vi "Example with Results.vi"(3 "Table Content":T1={"TableHeader"=["Soll\nppm/%", "Ist\nppm/%", "Fehler\n%", "Toleranz\n%", "Ergebnis"], "Table"=[["aaa", "bbb", "ccc", "ddd"], ["111", "222", "333", "444"], ["sss", "fff", "kkk", "xxx"], ["6.5", "11.13", "19.2", "4"], ["1111", "1212", "777", "888"]], "Relative Column Widths (%)"=[22.5, 22.5, 22.5, 22.5, 10.0], "Results"=[{"Result Text"="ok", "Result"=TRUE}, {"Result Text"="ko", "Result"=FALSE}, {"Result Text"="ko", "Result"=FALSE}, {"Result Text"="ok", "Result"=TRUE}, {"Result Text"="ok", "Result"=TRUE}], "PositionBemerkung"=enum."before", "PageBreak"=enum."before"}) -> (11 "XY-Graph":cluster{"X":dbl, "Y":dbl}[](graph))   [LabVIEW 2020, in "PDF Interface.lvlib"]
uses:
  PDF Interface.lvlib
  <vilib>/Simplicity AI/SAI_PDF_API/Classes/Context/Controls/SAI_PDF_Text Align.ctl
  <vilib>/Simplicity AI/SAI_PDF_API/Classes/Context/Context.lvclass
  <vilib>/Simplicity AI/SAI_PDF_API/Classes/Context/Controls/SAI_PDF_PDF Details.ctl
  PDF Interface Helper/PDFTableContentType.ctl
  PDF Interface Helper/PDF Interface Helper.lvlib
  PDF Interface Helper/PDFContentType.ctl
  PDF Interface Helper/PDFPageBreak.ctl
  PDF Interface Helper/PDFCommentPosition.ctl
  PDF Interface Helper/PDFTablePictures.ctl
  PDF Interface Helper/PDFResultPictures.ctl
  PDF Interface Helper/PDFResults.ctl
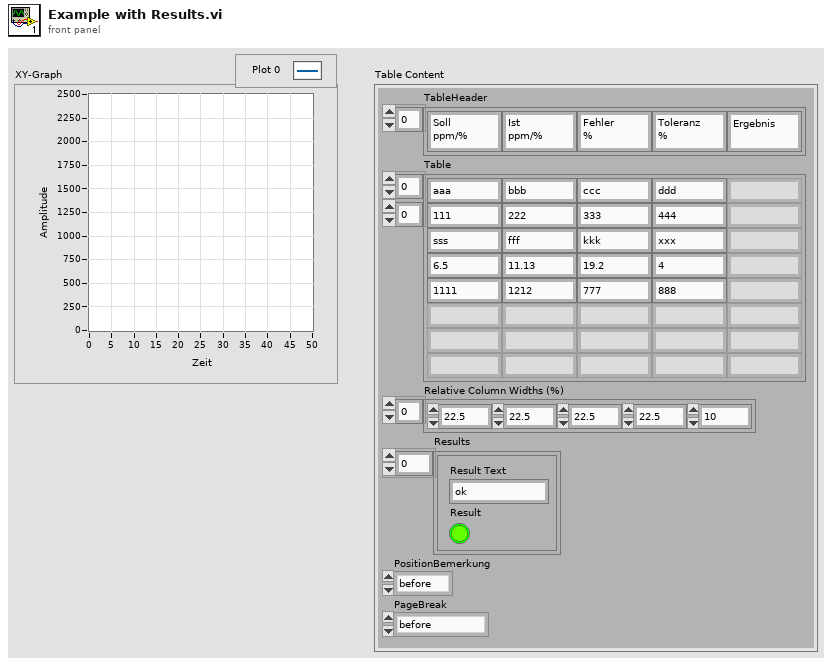
[diagram p1: front panel]
types:
  T1 = typedef "PDF Interface.lvlib/PDF Interface Helper.lvlib/PDFTableContentType.ctl" = cluster{"TableHeader":string[], "Table":string[][], "Relative Column Widths (%)":sgl[], "Results":cluster{"Result Text":string, "Result":bool}[], "PositionBemerkung":T2, "PageBreak":T3}
  T2 = typedef "PDF Interface.lvlib/PDF Interface Helper.lvlib/PDFCommentPosition.ctl" = enum16{"before", "after"}
  T3 = typedef "PDF Interface.lvlib/PDF Interface Helper.lvlib/PDFPageBreak.ctl" = enum16{"none", "before", "after", "after comment"}
  T4 = typedef "PDF Interface.lvlib/PDF Interface Helper.lvlib/PDFContentType.ctl" = cluster{"Titel":string, "Header Table":string[][], "Table Array":T5[], "Bemerkungen":cluster{"Bemerkung Text":string, "Align (Left)":T9, "Add Line Feeds (F:No)":bool}[]}
  T5 = typedef "PDF Interface.lvlib/PDF Interface Helper.lvlib/PDFTableContentType.ctl" = cluster{"TableHeader":string[], "Table":string[][], "Relative Column Widths (%)":sgl[], "Results":T6, "PositionBemerkung":T2, "PageBreak":T3, "TablePictures":T8, "Horizontal Align":i32}
  T6 = typedef "PDF Interface.lvlib/PDF Interface Helper.lvlib/PDFResults.ctl" = cluster{"Results":cluster{"Result Text":string, "Result":bool}[], "ResultPictures":T7, "use Pictures":bool}
  T7 = typedef "PDF Interface.lvlib/PDF Interface Helper.lvlib/PDFResultPictures.ctl" = cluster{"Yes Ctl Refnum":refnum<vi>, "No Ctl Refnum":refnum<vi>}
  T8 = typedef "PDF Interface.lvlib/PDF Interface Helper.lvlib/PDFTablePictures.ctl" = cluster{"Ctl Refnum In":refnum<vi>[], "RowOrColumn":enum16{"Row", "Column"}, "IndexToInsert":u16, "Image Scale (%)":sgl[], "Autoscale? (T)":bool[], "Horizontal Align":i32}
  T9 = typedef "SAI_PDF_Toolkit.lvlib/Context.lvclass/SAI_PDF_Text Align.ctl" = i32
  T10 = cluster{"Bemerkung Text":string, "Align (Left)":T9, "Add Line Feeds (F:No)":bool}[]
  T11 = cluster{"GraphCtl Refnum":refnum<vi>, "Wrap Text (F:No)":bool, "Hide Grid (F:No)":bool, "Scale (100%)":sgl, "Align (Left)":T9}
  T12 = typedef "SAI_PDF_Toolkit.lvlib/Context.lvclass/SAI_PDF_PDF Details.ctl" = cluster{"Title":string, "Subject":string, "Keywords":string, "Author":string, "Creator":string}
  T13 = cluster{"Header Footer Text Cluster":cluster{"Header Text":string, "Footer Text":string, "Time":string, "Page Number":string}, "PDF Details":T12}
  T14 = cluster{"GraphCtl Refnum":refnum<vi>, "Wrap Text (F:No)":bool, "Hide Grid (F:No)":bool, "Scale (100%)":sgl, "Align (Left)":T9}[]
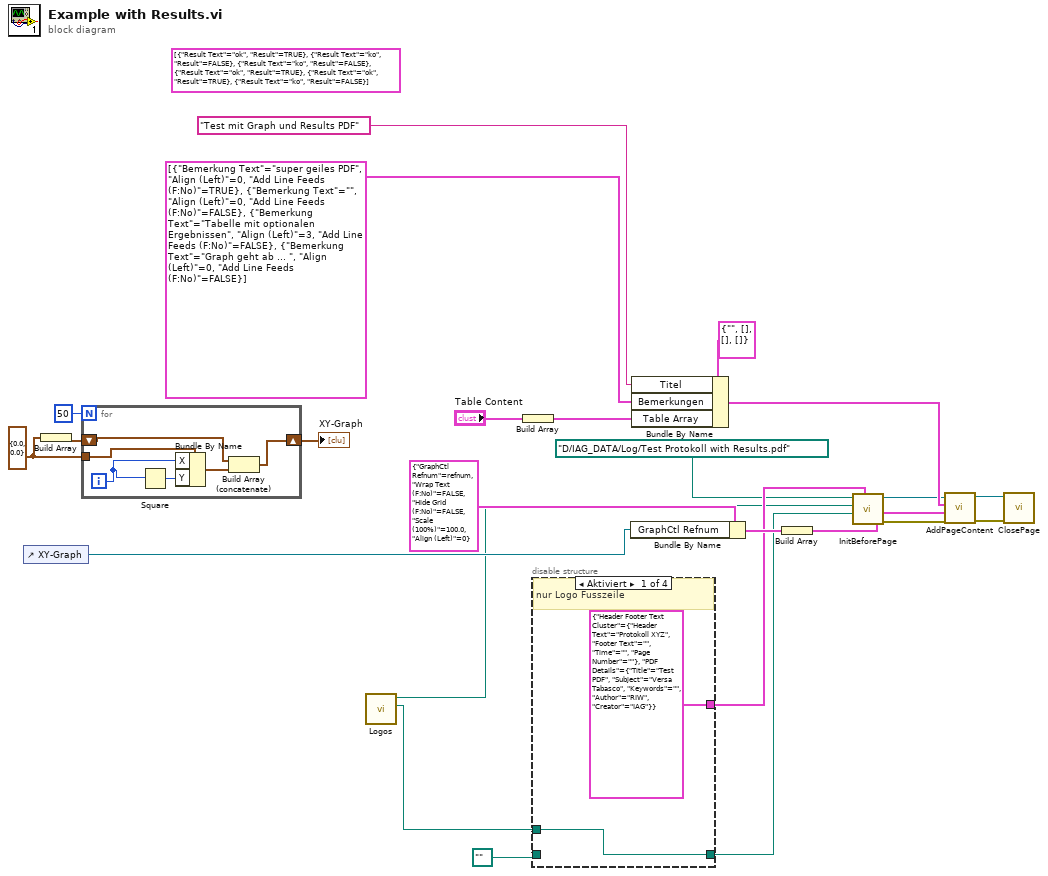
[diagram p0: block diagram]
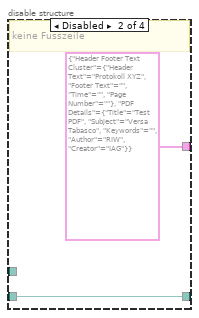
[diagram p2: hidden frame]
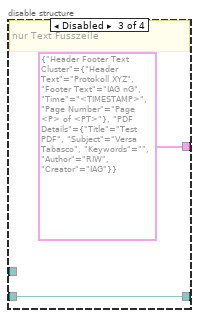
[diagram p3: hidden frame]
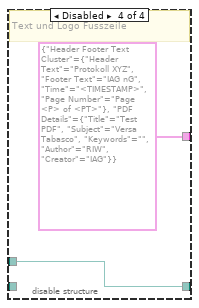
[diagram p4: hidden frame]
diagram:
  (unwired) cluster{"Result Text":string, "Result":bool}[] [{"Result Text"="ok", "Result"=TRUE}, {"Result Text"="ko", "Result"=FALSE}, {"Result Text"="ko", "Result"=FALSE}, {"Result Text"="ok", "Result"=TRUE}, {"Result Text"="ok", "Result"=TRUE}, {"Result Text"="ko", "Result"=FALSE}] ("Results")
  w21 = cluster{"X":dbl, "Y":dbl} {"X"=0.0, "Y"=0.0} ("XY-Graph")
  n1 = control-ref of="XY-Graph"() -> (w18:refnum<vi>)
  n2 = Build Array(w21) -> (w22:cluster{"X":dbl, "Y":dbl}[])
  n3 = for {
    N: 50 -> [_]
    shift-right: [w25] -> w23
    shift-left: w22 -> [w27]
    tunnel: w21 -> [w26]
    i -> [w29]
    n4 = Square(x=w29) -> (x^2=w30:i32)
    n5 = Bundle By Name(cluster=w26, "X"=w29, "Y"=w30) -> (w28:cluster{"X":dbl, "Y":dbl})
    n6 = Build Array (concatenate)(w27, w28) -> (w25:cluster{"X":dbl, "Y":dbl}[])
  }
  "XY-Graph" <- w23
  n7 = call "Logos.vi"() -> ("Footer Image File Path"=w13:path, "Header Image File Path"=w10:path)  [unwired: 9 in, 1 out]
  n8 = Build Array("Table Content") -> (w1:T1[])
  n9 = disable-structure shown="Aktiviert" {
    disable-tunnel: [T13 {"Header Footer Text Cluster"={"Header Text"="Protokoll XYZ", "Footer Text"="", "Time"="", "Page Number"=""}, "PDF Details"={"Title"="Test PDF", "Subject"="Versa Tabasco", "Keywords"="", "Author"="RIW", "Creator"="IAG"}} ("Info") T13 {"Header Footer Text Cluster"={"Header Text"="Protokoll XYZ", "Footer Text"="", "Time"="", "Page Number"=""}, "PDF Details"={"Title"="Test PDF", "Subject"="Versa Tabasco", "Keywords"="", "Author"="RIW", "Creator"="IAG"}} ("Info") T13 {"Header Footer Text Cluster"={"Header Text"="Protokoll XYZ", "Footer Text"="IAG nG", "Time"="<TIMESTAMP>", "Page Number"="Page <P> of <PT>"}, "PDF Details"={"Title"="Test PDF", "Subject"="Versa Tabasco", "Keywords"="", "Author"="RIW", "Creator"="IAG"}} ("Info") T13 {"Header Footer Text Cluster"={"Header Text"="Protokoll XYZ", "Footer Text"="IAG nG", "Time"="<TIMESTAMP>", "Page Number"="Page <P> of <PT>"}, "PDF Details"={"Title"="Test PDF", "Subject"="Versa Tabasco", "Keywords"="", "Author"="RIW", "Creator"="IAG"}} ("Info")] -> w12
    disable-tunnel: w13 -> [w31 _ _ w37]
    disable-tunnel: path "" ("Footer Image File Path") -> [_ w33 w35 _]
    disable-tunnel: [w31 w33 w35 w37] -> w9
    frame Enabled {
      # "nur Logo Fusszeile"
    }
    frame Disabled {
      # "keine Fusszeile"
    }
    frame Disabled {
      # "nur Text Fusszeile"
    }
    frame Disabled {
      # "Text und Logo Fusszeile"
    }
  }
  n10 = Bundle By Name(cluster=T11 {"GraphCtl Refnum"=refnum, "Wrap Text (F:No)"=FALSE, "Hide Grid (F:No)"=FALSE, "Scale (100%)"=100.0, "Align (Left)"=0} ("Graph"), "GraphCtl Refnum"=w18) -> (w19:T11)
  n11 = Bundle By Name(cluster=T4 {"Titel"="", "Header Table"=[], "Table Array"=[], "Bemerkungen"=[]} ("Content"), "Titel"="Test mit Graph und Results PDF", "Bemerkungen"=T10 [{"Bemerkung Text"="super geiles PDF", "Align (Left)"=0, "Add Line Feeds (F:No)"=TRUE}, {"Bemerkung Text"="", "Align (Left)"=0, "Add Line Feeds (F:No)"=FALSE}, {"Bemerkung Text"="Tabelle mit optionalen Ergebnissen", "Align (Left)"=3, "Add Line Feeds (F:No)"=FALSE}, {"Bemerkung Text"="Graph geht ab ... ", "Align (Left)"=0, "Add Line Feeds (F:No)"=FALSE}], "Table Array"=w1) -> (w8:T4)
  n12 = Build Array(w19) -> (w3:T14)
  n13 = call "InitBeforePage.vi"("Info"=w12, "Footer Image File Path"=w9, "Header Image File Path"=w10, "Path (Dialog if Empty)"=path "D:/IAG_DATA/Log/Test Protokoll with Results.pdf") -> ("Fehler (Ausgang)"=w7:errorcluster, "Context (Ausgang)"=w6:refnum<class "Context.lvclass">)  [unwired: 6 in]
  n14 = call "AddPageContent.vi"("error in"=w7, "Graph Array"=w3, "Content"=w8, "Context (Eingang)"=w6) -> ("error out"=w5:errorcluster, "Context (Ausgang)"=w4:refnum<class "Context.lvclass">)  [unwired: 6 in]
  n15 = call "ClosePage.vi"("Fehler (Eingang, kein Fehler)"=w5, "Context (Eingang)"=w4) -> ()  [unwired: 9 in, 1 out]
